vi "detect_goal.vi"(0 "Image Out":T1) -> (1 "goal_pos":cluster{"ave x":dbl, "ave y":dbl}[](array[cluster]), 2 "X Resolution":i32, 3 "Y Resolution":i32)   [LabVIEW 2018]
uses:
  <vilib>/vision/Image Controls.llb/IMAQ Image.ctl
  <vilib>/vision/Measure.llb/Edge Options.ctl
  <vilib>/vision/Measure.llb/Edge Polarity.ctl
  <vilib>/vision/NI_Vision_Development_Module.lvlib
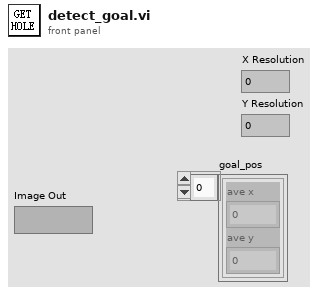
[diagram p1: front panel]
types:
  T1 = typedef "IMAQ Image.ctl" = refnum<image>
  T2 = typedef "Edge Options.ctl" = cluster{"Edge Polarity":T3, "Kernel Size":u32, "Width":u32, "Minimum Edge Strength":sgl, "Interpolation Type":enum32{"Zero Order", "Bilinear", "Quadratic", "Cubic", "Bilinear Fixed"}, "Data Processing Method":enum32{"Average", "Median"}}
  T3 = typedef "Edge Polarity.ctl" = u32
  T4 = cluster{"Search Direction":u32, "Edge Options":T2, "Show Search Area":bool, "Show Search Lines":bool, "Show Edges Found":bool, "Show Result":bool, "Search Area Color":u32, "Search Lines Color":u32, "Edge Locations Color":u32, "Result Color":u32, "Overlay Group Name":string}
  T5 = typedef "ROI Descriptor" = cluster{"Global Rectangle":i32[], "Contours":cluster{"ID":enum32{"External", "Internal"}, "Type":u32, "Coordinates":i32[]}[]}
  T6 = cluster{"Point1 (Pixels)":cluster{"X":sgl, "Y":sgl}, "Point2 (Pixels)":cluster{"X":sgl, "Y":sgl}, "Point1 (Real-World)":cluster{"X":sgl, "Y":sgl}, "Point2 (Real-World)":cluster{"X":sgl, "Y":sgl}, "Angle (Pixel)":dbl, "Angle (Real-World)":dbl, "Score":dbl, "Straightness":dbl, "Average SNR (db)":dbl, "Calibration Valid":bool}[]
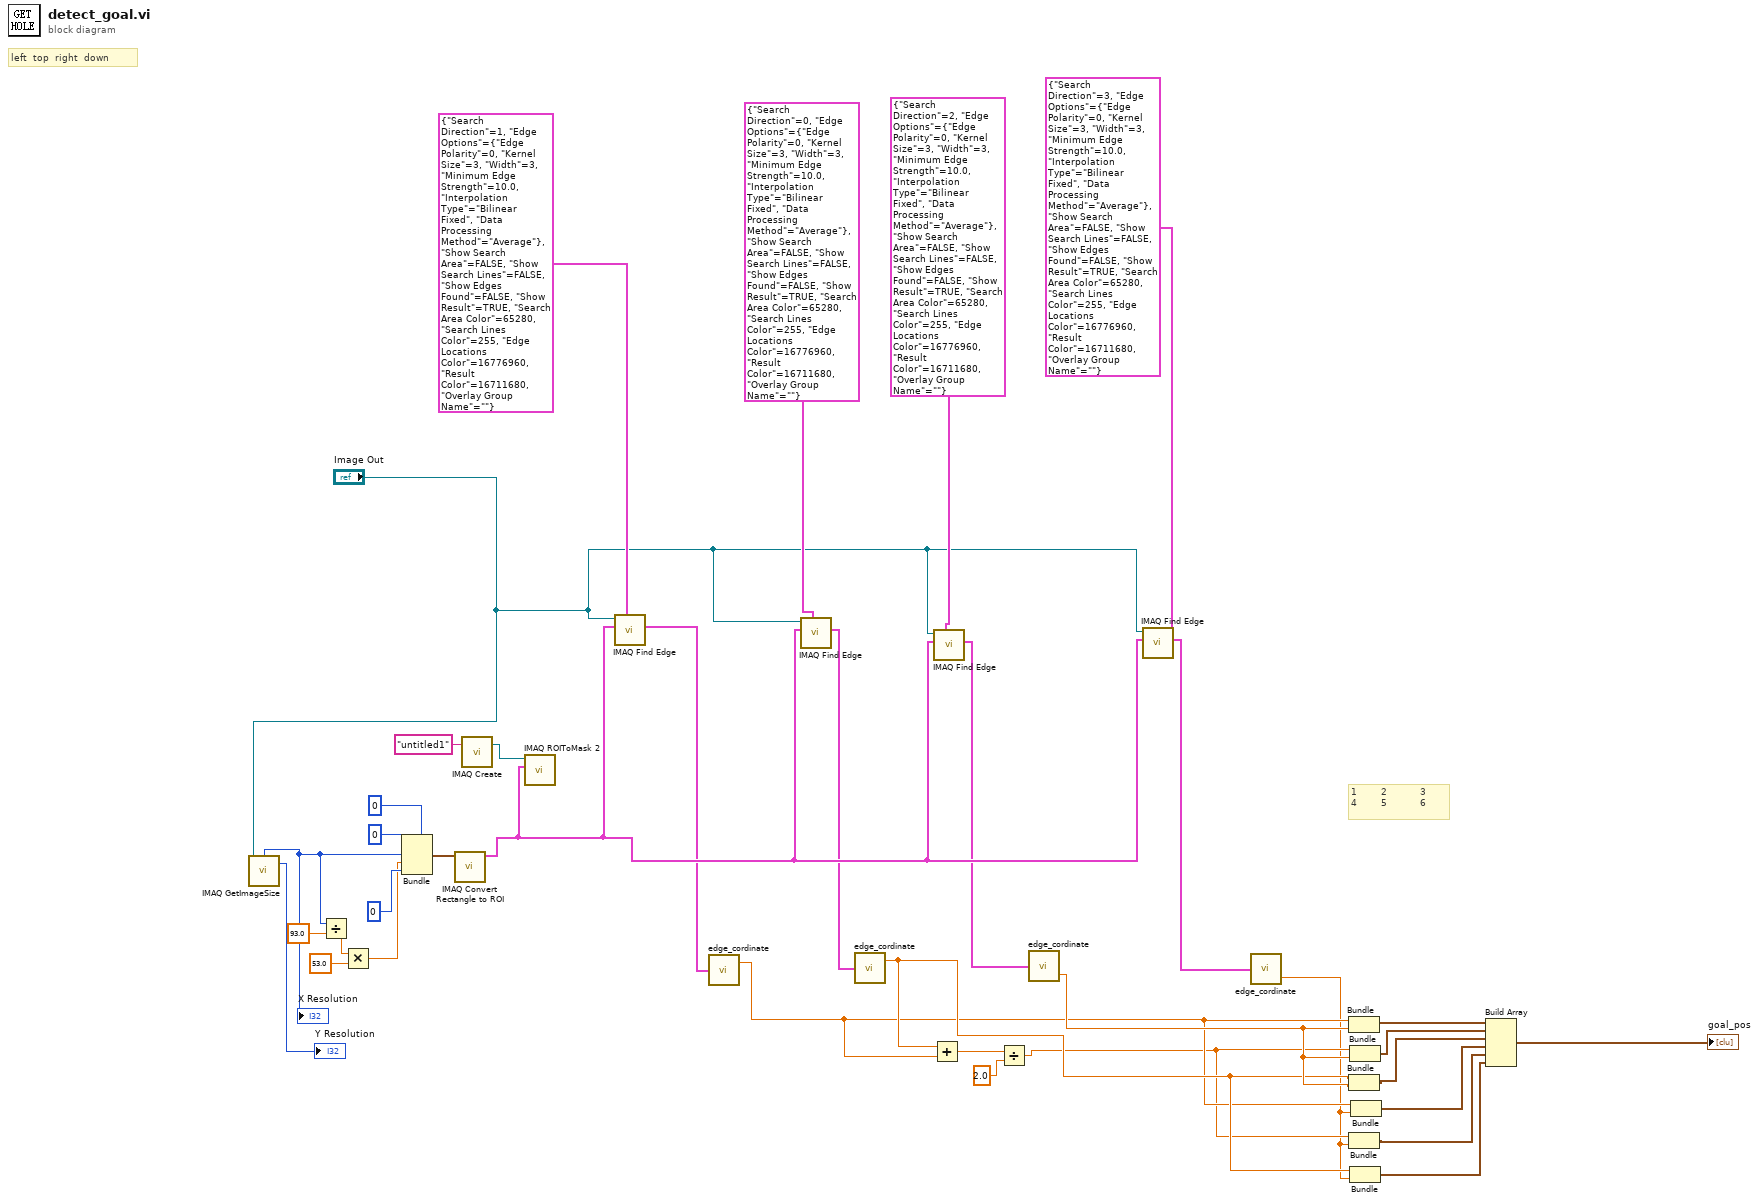
[diagram p0: block diagram]
diagram:
  # "1        2           3\n4        5           6"
  # "left  top  right  down"
  n1 = call "IMAQ GetImageSize"("Image"="Image Out") -> ("Y Resolution"=→"Y Resolution":i32, "X Resolution"=w5:i32)  [unwired: 3 in, 1 out]
  "X Resolution" <- w5
  n2 = Divide(x=w5, y=93.0) -> (x/y=w4:dbl)
  n3 = Multiply(x=w4, y=53.0) -> (x*y=w2:dbl)
  n4 = Bundle(0, 0, "X Resolution"=w5, w2, 0) -> (w31:cluster{i32, i32, "X Resolution":i32, dbl, i32})  [unwired: 1 in]
  n5 = call "IMAQ Convert Rectangle to ROI"("Rectangle"=w31) -> ("ROI Descriptor"=w30:T5)  [unwired: 8 in, 1 out]
  n6 = call "IMAQ Create"("Image Name"="untitled1") -> ("New Image"=w29:T1)  [unwired: 4 in, 1 out]
  n7 = call "IMAQ ROIToMask 2"("ROI Descriptor"=w30, "Image"=w29) -> ()  [unwired: 7 in, 3 out]
  n8 = call "IMAQ Find Edge"("Options"=T4 {"Search Direction"=1, "Edge Options"={"Edge Polarity"=0, "Kernel Size"=3, "Width"=3, "Minimum Edge Strength"=10.0, "Interpolation Type"=enum."Bilinear Fixed", "Data Processing Method"=enum."Average"}, "Show Search Area"=FALSE, "Show Search Lines"=FALSE, "Show Edges Found"=FALSE, "Show Result"=TRUE, "Search Area Color"=65280, "Search Lines Color"=255, "Edge Locations Color"=16776960, "Result Color"=16711680, "Overlay Group Name"=""}, "ROI Descriptor"=w30, "Image"="Image Out") -> ("Straight Edges"=w25:T6)  [unwired: 5 in, 3 out]
  n9 = call "edge_cordinate.vi"("Straight Edges"=w25) -> ("ave x"=w13:dbl)  [unwired: 1 out]
  n10 = call "IMAQ Find Edge"("Options"=T4 {"Search Direction"=0, "Edge Options"={"Edge Polarity"=0, "Kernel Size"=3, "Width"=3, "Minimum Edge Strength"=10.0, "Interpolation Type"=enum."Bilinear Fixed", "Data Processing Method"=enum."Average"}, "Show Search Area"=FALSE, "Show Search Lines"=FALSE, "Show Edges Found"=FALSE, "Show Result"=TRUE, "Search Area Color"=65280, "Search Lines Color"=255, "Edge Locations Color"=16776960, "Result Color"=16711680, "Overlay Group Name"=""}, "ROI Descriptor"=w30, "Image"="Image Out") -> ("Straight Edges"=w24:T6)  [unwired: 5 in, 3 out]
  n11 = call "edge_cordinate.vi"("Straight Edges"=w24) -> ("ave x"=w15:dbl)  [unwired: 1 out]
  n12 = Add(x=w15, y=w13) -> (x+y=w20:dbl)
  n13 = call "IMAQ Find Edge"("Options"=T4 {"Search Direction"=2, "Edge Options"={"Edge Polarity"=0, "Kernel Size"=3, "Width"=3, "Minimum Edge Strength"=10.0, "Interpolation Type"=enum."Bilinear Fixed", "Data Processing Method"=enum."Average"}, "Show Search Area"=FALSE, "Show Search Lines"=FALSE, "Show Edges Found"=FALSE, "Show Result"=TRUE, "Search Area Color"=65280, "Search Lines Color"=255, "Edge Locations Color"=16776960, "Result Color"=16711680, "Overlay Group Name"=""}, "ROI Descriptor"=w30, "Image"="Image Out") -> ("Straight Edges"=w23:T6)  [unwired: 5 in, 3 out]
  n14 = Divide(x=w20, y=2.0) -> (x/y=w11:dbl)
  n15 = call "edge_cordinate.vi"("Straight Edges"=w23) -> ("ave y"=w17:dbl)  [unwired: 1 out]
  n16 = call "IMAQ Find Edge"("Options"=T4 {"Search Direction"=3, "Edge Options"={"Edge Polarity"=0, "Kernel Size"=3, "Width"=3, "Minimum Edge Strength"=10.0, "Interpolation Type"=enum."Bilinear Fixed", "Data Processing Method"=enum."Average"}, "Show Search Area"=FALSE, "Show Search Lines"=FALSE, "Show Edges Found"=FALSE, "Show Result"=TRUE, "Search Area Color"=65280, "Search Lines Color"=255, "Edge Locations Color"=16776960, "Result Color"=16711680, "Overlay Group Name"=""}, "ROI Descriptor"=w30, "Image"="Image Out") -> ("Straight Edges"=w22:T6)  [unwired: 5 in, 3 out]
  n17 = call "edge_cordinate.vi"("Straight Edges"=w22) -> ("ave y"=w10:dbl)  [unwired: 1 out]
  n18 = Bundle("ave x"=w13, "ave y"=w17) -> (w21:cluster{"ave x":dbl, "ave y":dbl})  [unwired: 1 in]
  n19 = Bundle("ave x"=w15, "ave y"=w17) -> (w16:cluster{"ave x":dbl, "ave y":dbl})  [unwired: 1 in]
  n20 = Bundle(w11, "ave y"=w10) -> (w9:cluster{dbl, "ave y":dbl})  [unwired: 1 in]
  n21 = Bundle(w11, "ave y"=w17) -> (w18:cluster{dbl, "ave y":dbl})  [unwired: 1 in]
  n22 = Bundle("ave x"=w15, "ave y"=w10) -> (w14:cluster{"ave x":dbl, "ave y":dbl})  [unwired: 1 in]
  n23 = Bundle("ave x"=w13, "ave y"=w10) -> (w12:cluster{"ave x":dbl, "ave y":dbl})  [unwired: 1 in]
  n24 = Build Array(w21, w18, w16, w12, w9, w14) -> (→"goal_pos":cluster{"ave x":dbl, "ave y":dbl}[])
